vi "Evaluate Sleep Request.vi"(1 "String In":string) -> (0 "Test OK":bool)   [LabVIEW 2022 SP3]
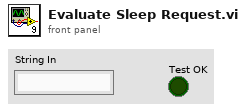
[diagram p1: front panel]
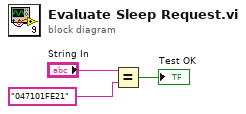
[diagram p0: block diagram]
diagram:
  n1 = Equal?(x="String In", y="047101FE21") -> (x = y?=→"Test OK":bool)
